vi "Configure Capacitance.vi"(0 "VISA resource name":refnum<visa-resource-name>, 5 "error in (no error)":errorcluster, 6 "Auto Range? (T: Auto)":bool=TRUE, 7 "Digital Filter (0: Off)":u16(ring) items=["Off", "Moving Filter", "Repeating Filter"], 8 "Range":u16(ring) items=["1 nF", "10 nF", "100 nF", "1 uF", "10 uF", "100 uF", "1 mF", "10 mF"], 9 "Digital Filter Readings (10)":i32=10, 10 "Function":i32(ring) items=["Primary", "Secondary"]) -> (14 "VISA resource name out":refnum<visa-resource-name>, 19 "error out":errorcluster)   [LabVIEW 2020, in "Keithley 2100 Series.lvlib"]
doc: "This VI configures the instrument to measure Capacitance.\n\nThis Vi will not support KE2100."
uses:
  Keithley 2100 Series.lvlib
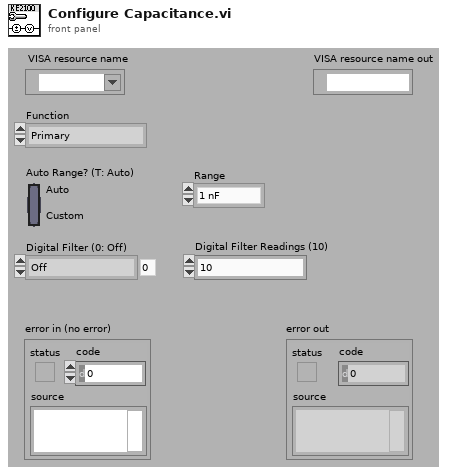
[diagram p1: front panel]
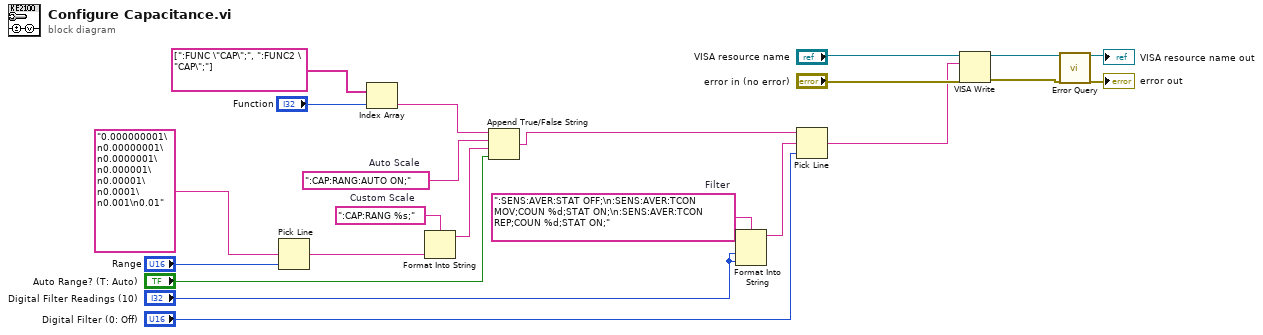
[diagram p0: block diagram]
diagram:
  w14 = ":SENS:AVER:STAT OFF;\n:SENS:AVER:TCON MOV;COUN %d;STAT ON;\n:SENS:AVER:TCON REP;COUN %d;STAT ON;"  # Filter
  w16 = ":CAP:RANG:AUTO ON;"  # Auto Scale
  w18 = ":CAP:RANG %s;"  # Custom Scale
  n1 = Pick Line(multi-line string="0.000000001\n0.00000001\n0.0000001\n0.000001\n0.00001\n0.0001\n0.001\n0.01", line index="Range") -> (output string=w4:string)  [unwired: 1 in]
  n2 = Index Array(array=string[] [":FUNC \"CAP\";", ":FUNC2 \"CAP\";"], index="Function") -> (element=w1:string)
  n3 = Format Into String(format string=w18, w4) -> (resulting string=w17:string)  [unwired: 2 in, 1 out]
  n4 = Append True/False String(1:"Auto Range? (T: Auto)", 2:w17, 3:w16, 4:w1) -> (0:w10:string)
  n5 = Format Into String(format string=w14, "Digital Filter Readings (10)", "Digital Filter Readings (10)") -> (resulting string=w15:string)  [unwired: 2 in, 1 out]
  n6 = Pick Line(string ("")=w10, multi-line string=w15, line index="Digital Filter (0: Off)") -> (output string=w9:string)
  n7 = VISA Write(VISA resource name="VISA resource name", write buffer=w9, error in (no error)="error in (no error)") -> (VISA resource name out=w8:refnum<visa-resource-name>, error out=w7:errorcluster)  [unwired: 1 out]
  n8 = call "Error Query.vi"("VISA resource name"=w8, "error in (no error)"=w7) -> ("VISA resource name out"=→"VISA resource name out":refnum<visa-resource-name>, "error out"=→"error out":errorcluster)  [unwired: 14 in, 2 out]
